vi "GlobalPlanner_Recycle_Msg.vi"(8 "error in (no error)":errorcluster caption="错误输入（无错误）", 10 "值(信号)":bool, 11 "GlobalPlanner输入":refnum<class "GlobalPlanner.lvclass">) -> (0 "error out":errorcluster caption="错误输出", 3 "GlobalPlanner输出":refnum<class "GlobalPlanner.lvclass">)   [LabVIEW 2014, in "GlobalPlanner.lvlib" / "GlobalPlanner.lvclass"]
uses:
  GlobalPlanner.lvclass
  GlobalPlanner.lvclass/GlobalPlanner.ctl
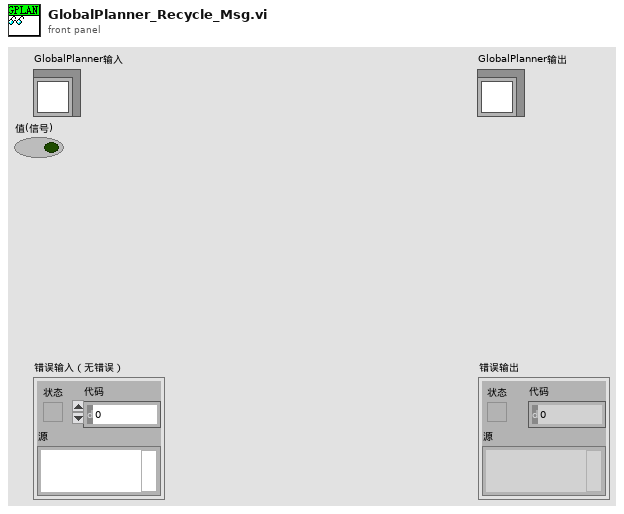
[diagram p1: front panel]
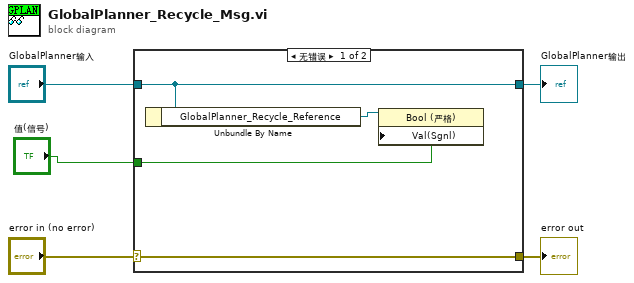
[diagram p0: block diagram]
diagram:
  n1 = case shown="无错误" "error in (no error)" {
    selector: "error in (no error)" -> [w9 w10]
    tunnel: [w9 w10] -> w4
    tunnel: [w8 w11] -> w2
    tunnel: "GlobalPlanner输入" -> [w8 w11]
    tunnel: "值(信号)" -> [w6 _]
    frame No Error {
      n2 = Unbundle By Name(w8) -> ("GlobalPlanner_Recycle_Reference"=w7:refnum<vi>)
      n3 = property class="Bool (严格)"(reference=w7, "Val(Sgnl)"=w6) -> ()  [unwired: 1 in, 2 out]
    }
    frame Error {
    }
  }
  "error out" <- w4
  "GlobalPlanner输出" <- w2
